vi "Print average graph.vi"(4 "Max cluster":T2 {"Hour" format="%<%H:%M>t"}, 5 "Min Cluster":T1 {"Hour" format="%<%H:%M>t"}, 6 "dates":string[](array[string]), 7 "Weekday filter":T3, 8 "Input selected file path":path, 9 "Peaks":dbl[](graph), 10 "%":dbl[](array[numeric]) format="%.2f", 11 "data 2":dbl[][](array[numeric])) -> (0 "selected file path":path)   [LabVIEW 2018]
panel:
  out "Days:":string
  out "To":string
  out "From":string
  out "G-6:15PM-8:00PM 2":dbl format="%.1f"
  out "H-8:15PM-10:00PM 2":dbl format="%.1f"
  out "F-4:15PM-6:00PM 2":dbl format="%.1f"
  out "E-2:15PM-4:00PM 2":dbl format="%.1f"
  out "D-12:15 -2:00PM 2":dbl format="%.1f"
  out "C-10:15-12:00 2":dbl format="%.1f"
  out "B-8:15-10:00 2":dbl format="%.1f"
  out "A-6:15-8:00 2":dbl format="%.1f"
  out "Peaks 2":dbl[](graph)
  out "Average usage":dbl[][](graph)
  # "```"
  # "PEAKS"
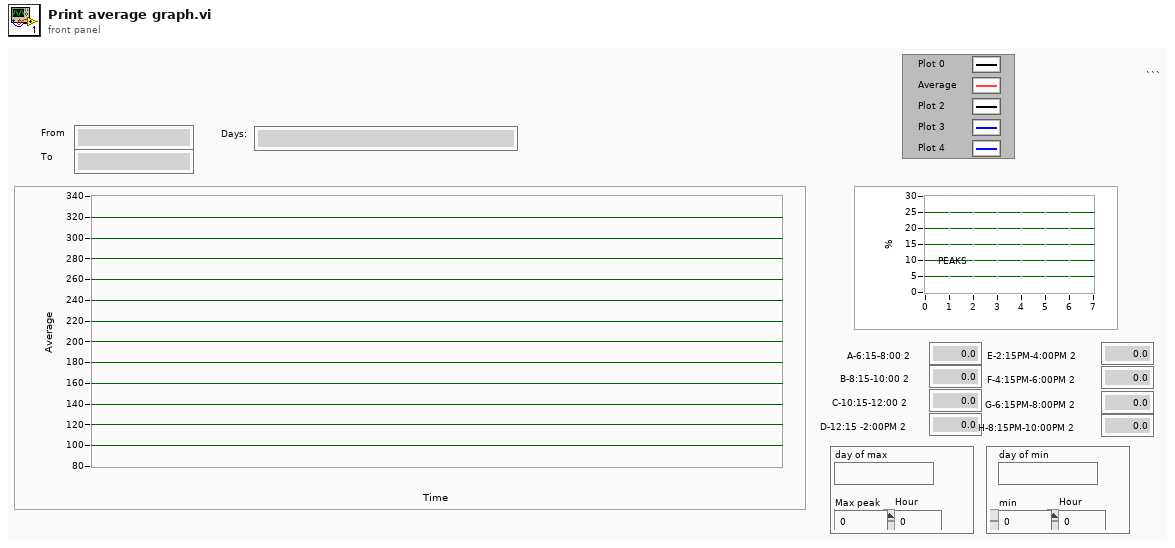
[diagram p1: front panel]
types:
  T1 = cluster{"Hour":i32, "min":dbl, "day of min":string}
  T2 = cluster{"Hour":i32, "Max peak":dbl, "day of max":string}
  T3 = cluster{"Monday":bool, "Tuesday":bool, "Wednesday":bool, "Thursday":bool, "Friday":bool, "Saturday":bool, "Sunday":bool}
  T4 = enum32{"Custom", "Standard", "Using Panel", "Using SubVI", "Complete"}
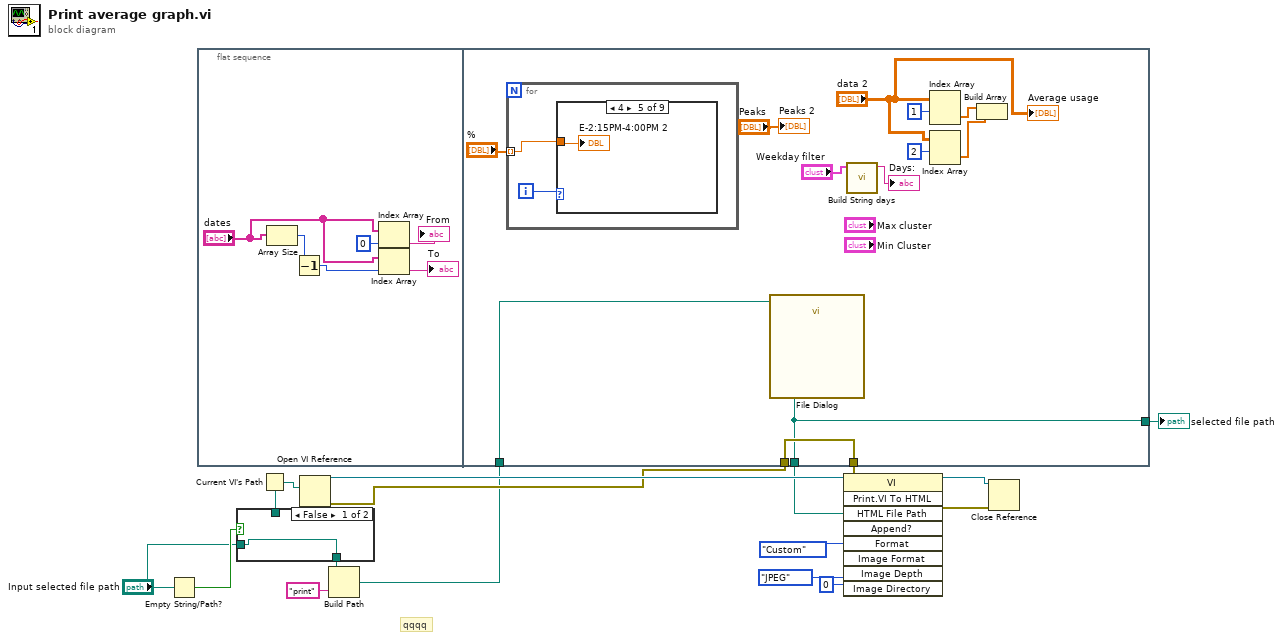
[diagram p0: block diagram]
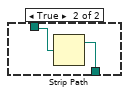
[diagram p2: hidden frame]
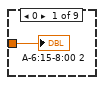
[diagram p3: hidden frame]
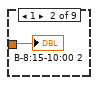
[diagram p4: hidden frame]
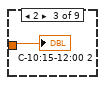
[diagram p5: hidden frame]
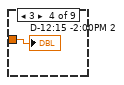
[diagram p6: hidden frame]
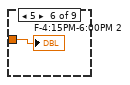
[diagram p7: hidden frame]
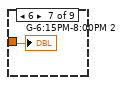
[diagram p8: hidden frame]
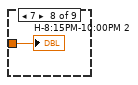
[diagram p9: hidden frame]
diagram:
  # "qqqq"
  n1 = Empty String/Path?(string/path="Input selected file path") -> (empty?=w2:bool)
  n2 = flat-sequence {
    tunnel: w8 -> [w34]
    tunnel: [w34] -> w7
    tunnel: w6 -> [w31]
    tunnel: [w23] -> w5
    tunnel: [w23] -> w3
    frame #0 {
      n3 = Array Size(array="dates") -> (size(s)=w20:i32)
      n4 = Decrement(x=w20) -> (x-1=w21:i32)
      n5 = Index Array(array="dates", index=0) -> (element=→"From":string)
      n6 = Index Array(array="dates", index=w21) -> (element=→"To":string)
    }
    frame #1 {
      n7 = for {
        tunnel: "%" -> [w36] mode=indexing
        i -> [w35]
        n8 = case shown="4" w35 {
          tunnel: w36 -> [w37 w38 w39 w40 w41 w42 w43 w44 _]
          frame 0 {
            "A-6:15-8:00 2" <- w37
          }
          frame 1 {
            "B-8:15-10:00 2" <- w38
          }
          frame 2 {
            "C-10:15-12:00 2" <- w39
          }
          frame 3 {
            "D-12:15 -2:00PM 2" <- w40
          }
          frame 4 {
            "E-2:15PM-4:00PM 2" <- w41
          }
          frame 5 {
            "F-4:15PM-6:00PM 2" <- w42
          }
          frame 6 {
            "G-6:15PM-8:00PM 2" <- w43
          }
          frame 7 {
            "H-8:15PM-10:00PM 2" <- w44
          }
          frame 8, Default {
          }
        }
      }
      n9 = call "File Dialog"("start path"=w31) -> ("selected path"=w23:path)  [unwired: 11 in, 3 out]
      n10 = call "Build String days.vi"("Weekday filter"="Weekday filter") -> ("output string"=→"Days:":string)  [unwired: 10 in]
      n11 = Index Array(array="data 2", index (row)=1) -> (element=w26:dbl[])  [unwired: 1 in]
      n12 = Index Array(array="data 2", index (row)=2) -> (element=w25:dbl[])  [unwired: 1 in]
      n13 = Build Array(w26, w25) -> ()  [unwired: 1 out]
      "Average usage" <- "data 2"
      "Peaks 2" <- "Peaks"
    }
  }
  n14 = Current VI's Path() -> (path=w11:path)
  n15 = case shown="False" w2 {
    tunnel: w11 -> [_ w47]
    tunnel: [w45 w46] -> w10
    tunnel: "Input selected file path" -> [w45 _]
    frame False {
    }
    frame True {
      n16 = Strip Path(path=w47) -> (stripped path=w46:path)  [unwired: 1 out]
    }
  }
  n17 = Open VI Reference(vi path=w11) -> (vi reference=w16:refnum<vi>, error out=w8:errorcluster)  [unwired: 5 in]
  n18 = Build Path(base path=w10, name or relative path="print") -> (appended path=w6:path)
  n19 = invoke class="VI" method="Print.VI To HTML"(reference=w16, error in=w7, "HTML File Path"=w5, "Format"=T4."Custom", "Image Format"=enum32{"PNG", "JPEG", "GIF"}."JPEG", "Image Depth"=0) -> (reference out=w15:refnum<vi>, error out=w14:errorcluster)  [unwired: 3 in, 7 out]
  n20 = Close Reference(reference=w15, error in (no error)=w14) -> ()  [unwired: 1 out]
  "selected file path" <- w3
